vi "Lift.vi"() -> ()   [LabVIEW 2025]
panel:
  out "Boolean":bool
  in  "Floor 4":bool
  out "Target_Pos":i32
  in  "Floor 2 Down":bool
  in  "Floor 1 Down":bool
  in  "Floor 3 up":bool
  in  "Floor 2 UP":bool
  out "Current_Pos":i32
  out "Up/Down":bool
  out "On/Off":bool
  in  "stop":bool
  out "Lift":bool
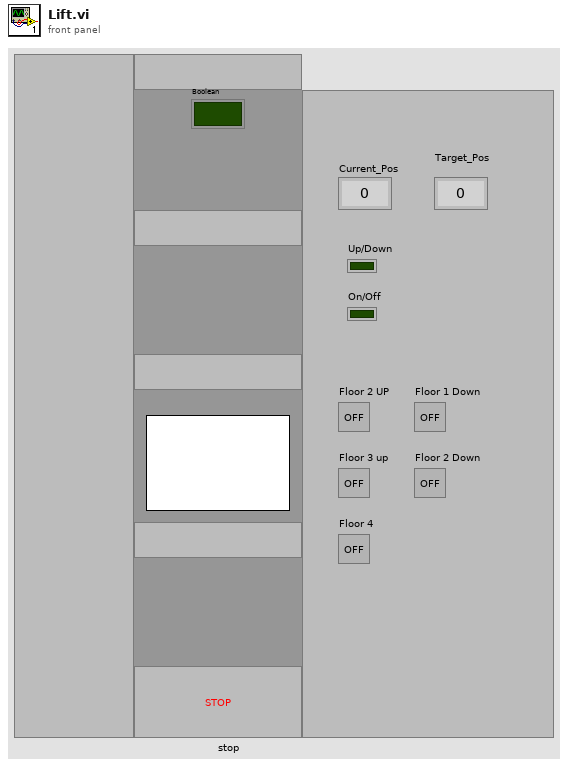
[diagram p1: front panel]
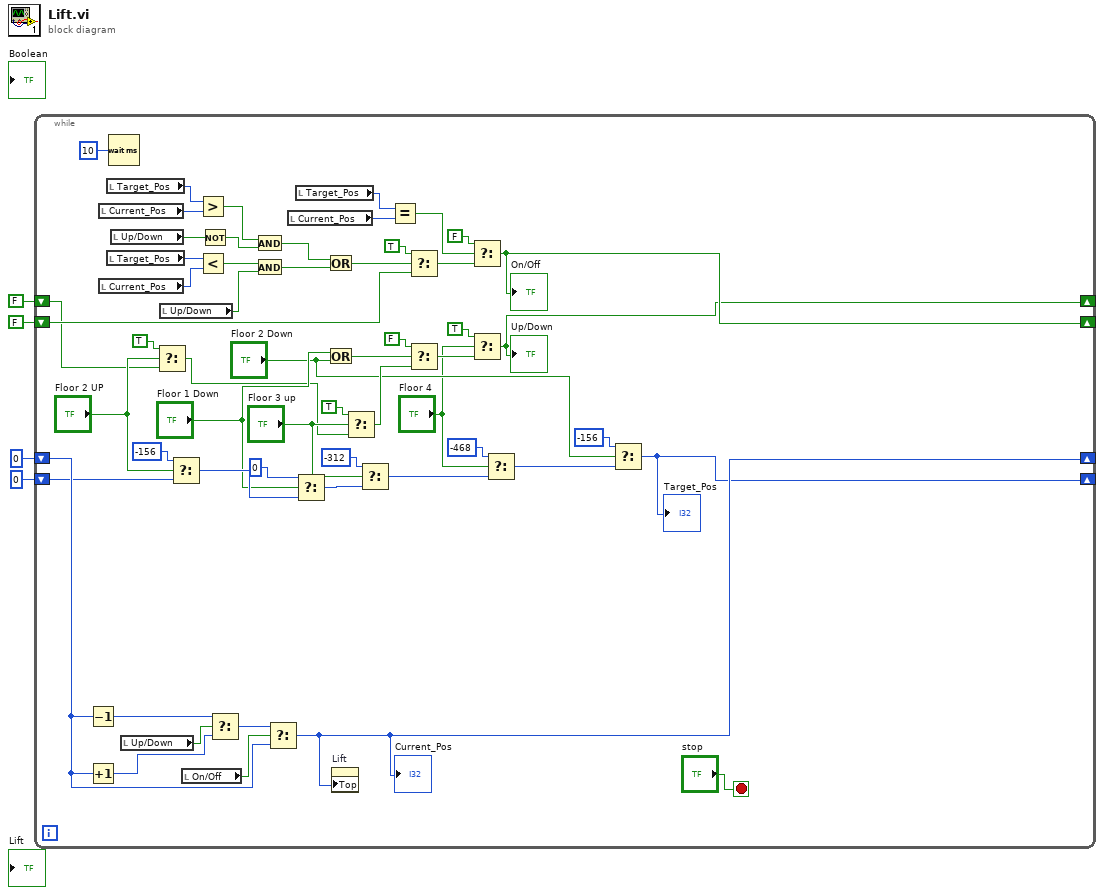
[diagram p0: block diagram]
diagram:
  n1 = while {
    shift-right: [w20] -> _
    shift-left: FALSE -> [w7]
    shift-right: [w54] -> _
    shift-left: 0 -> [w55]
    shift-right: [w44] -> _
    shift-left: FALSE -> [w51]
    shift-right: [w31] -> _
    shift-left: 0 -> [w34]
    stop <- "stop" stop-if-true
    n2 = Decrement(x=w55) -> (x-1=w58:i32)
    n3 = Increment(x=w55) -> (x+1=w57:i32)
    n4 = local read "Current_Pos"() -> (w15:i32)
    n5 = local read "Current_Pos"() -> (w45:i32)
    n6 = local read "Target_Pos"() -> (w16:i32)
    n7 = local read "Target_Pos"() -> (w46:i32)
    n8 = Wait (ms)(milliseconds to wait=u32 10) -> ()  [unwired: 1 out]
    n9 = local read "Up/Down"() -> (w13:bool)
    n10 = local read "Up/Down"() -> (w47:bool)
    n11 = Select(t=TRUE, s="Floor 2 UP", f=w7) -> (s? t:f=w5:bool)
    n12 = local read "Up/Down"() -> (w42:bool)
    n13 = Select(t=-156, s="Floor 2 UP", f=w34) -> (s? t:f=w33:i32)
    n14 = local read "On/Off"() -> (w53:bool)
    n15 = Greater?(x=w16, y=w15) -> (0:w14:bool)
    n16 = Less?(x=w46, y=w45) -> (x < y?=w43:bool)
    n17 = Not(x=w13) -> (.not. x?=w12:bool)
    n18 = Select(t=w58, s=w47, f=w57) -> (s? t:f=w56:i32)
    n19 = And(x=w14, y=w12) -> (x .and. y?=w10:bool)
    n20 = And(x=w43, y=w42) -> (x .and. y?=w41:bool)
    n21 = Select(t=w56, s=w53, f=w55) -> (s? t:f=w54:i32)
    "Current_Pos" <- w54
    n22 = local read "Current_Pos"() -> (w39:i32)
    n23 = local read "Target_Pos"() -> (w40:i32)
    n24 = Select(t=0, s="Floor 1 Down", f=w33) -> (s? t:f=w32:i32)
    n25 = Or(x=w10, y=w41) -> (x .or. y?=w11:bool)
    n26 = Or(x="Floor 1 Down", y="Floor 2 Down") -> (x .or. y?=w24:bool)
    n27 = property on="Lift" class="Bool (strict)"("Top"=w54) -> ()  [unwired: 2 in, 2 out]
    n28 = Select(t=TRUE, s="Floor 3 up", f=w5) -> (s? t:f=w37:bool)
    n29 = Select(t=-312, s="Floor 3 up", f=w32) -> (s? t:f=w23:i32)
    n30 = Equal?(x=w40, y=w39) -> (x = y?=w38:bool)
    n31 = Select(t=TRUE, s=w11, f=w51) -> (s? t:f=w50:bool)
    n32 = Select(t=FALSE, s=w24, f=w37) -> (s? t:f=w19:bool)
    n33 = Select(t=FALSE, s=w38, f=w50) -> (s? t:f=w44:bool)
    "On/Off" <- w44
    n34 = Select(t=TRUE, s="Floor 4", f=w19) -> (s? t:f=w20:bool)
    "Up/Down" <- w20
    n35 = Select(t=-468, s="Floor 4", f=w23) -> (s? t:f=w22:i32)
    n36 = Select(t=-156, s="Floor 2 Down", f=w22) -> (s? t:f=w31:i32)
    "Target_Pos" <- w31
  }
